vi "SCT Encode Type Descriptor.vi"(8 "error in (no error)":errorcluster, 11 "type descriptor":T1) -> (0 "error out":errorcluster, 3 "base64 encoded buffer":string)   [LabVIEW 2016]
uses:
  <vilib>/variable/Type Descriptor.ctl
  <vilib>/variable/NI_Variable.lvlib
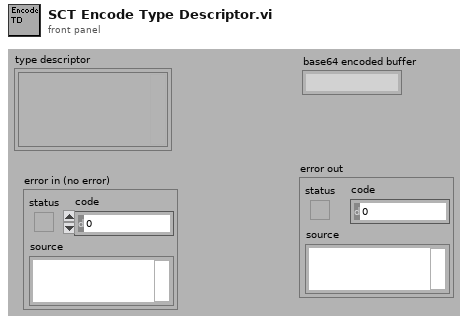
[diagram p1: front panel]
types:
  T1 = typedef "NI_Variable.lvlib/Type Descriptor.ctl" = cluster{"Variant":variant}
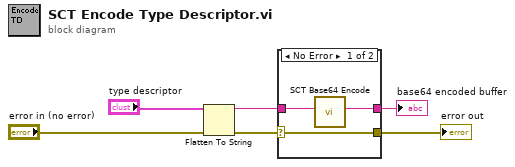
[diagram p0: block diagram]
diagram:
  n1 = Flatten To String(anything="type descriptor", error in (no error)="error in (no error)") -> (data string=w4:string, error out=w2:errorcluster)  [unwired: 2 in, 1 out]
  n2 = case shown="No Error" w2 {
    selector: w2 -> [w7 w10]
    tunnel: [w9 _] -> w6
    tunnel: w4 -> [w8 _]
    tunnel: [w7 w10] -> w1
    frame No Error {
      n3 = call <resource>:"SCT Base64 Encode.vi"("buffer in"=w8) -> ("base64 encoded buffer"=w9:string)  [unwired: 10 in]
    }
    frame Error {
    }
  }
  "base64 encoded buffer" <- w6
  "error out" <- w1
